vi "GradientSearchCoupling.vi"(0 "System no.":i32=1 min=1 max=4 step=1, 1 "Gradient Scan Names":string[](array[string]), 5 "error in (no error)":errorcluster) -> (19 "error out":errorcluster)   [LabVIEW 2020]
doc: "This VI allows to couple gradient search routines using the FRC command.\nAll changes are sent to the controller by pressing the OK button. If Cancel is selected or the window is closed, nothing will be sent to the controller."
uses:
  <vilib>/Utility/miscctls.llb/LVRowAndColumnTypeDef.ctl
  <vilib>/Utility/cursorutil.llb/Set Cursor (Icon Pict).vi
panel:
  in  "Gradient Search Routine Coupling":string[][](table)
  in  "OK Button":bool
  in  "Cancel Button":bool
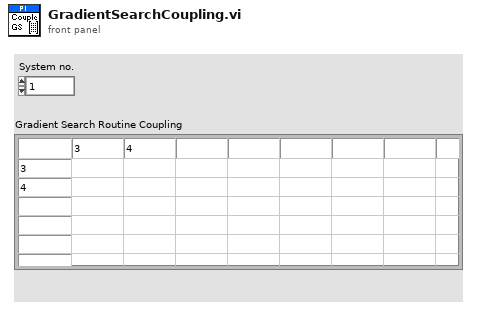
[diagram p1: front panel]
types:
  T1 = typedef "LVRowAndColumnTypeDef.ctl" = cluster{"Row":i32, "Column":i32}
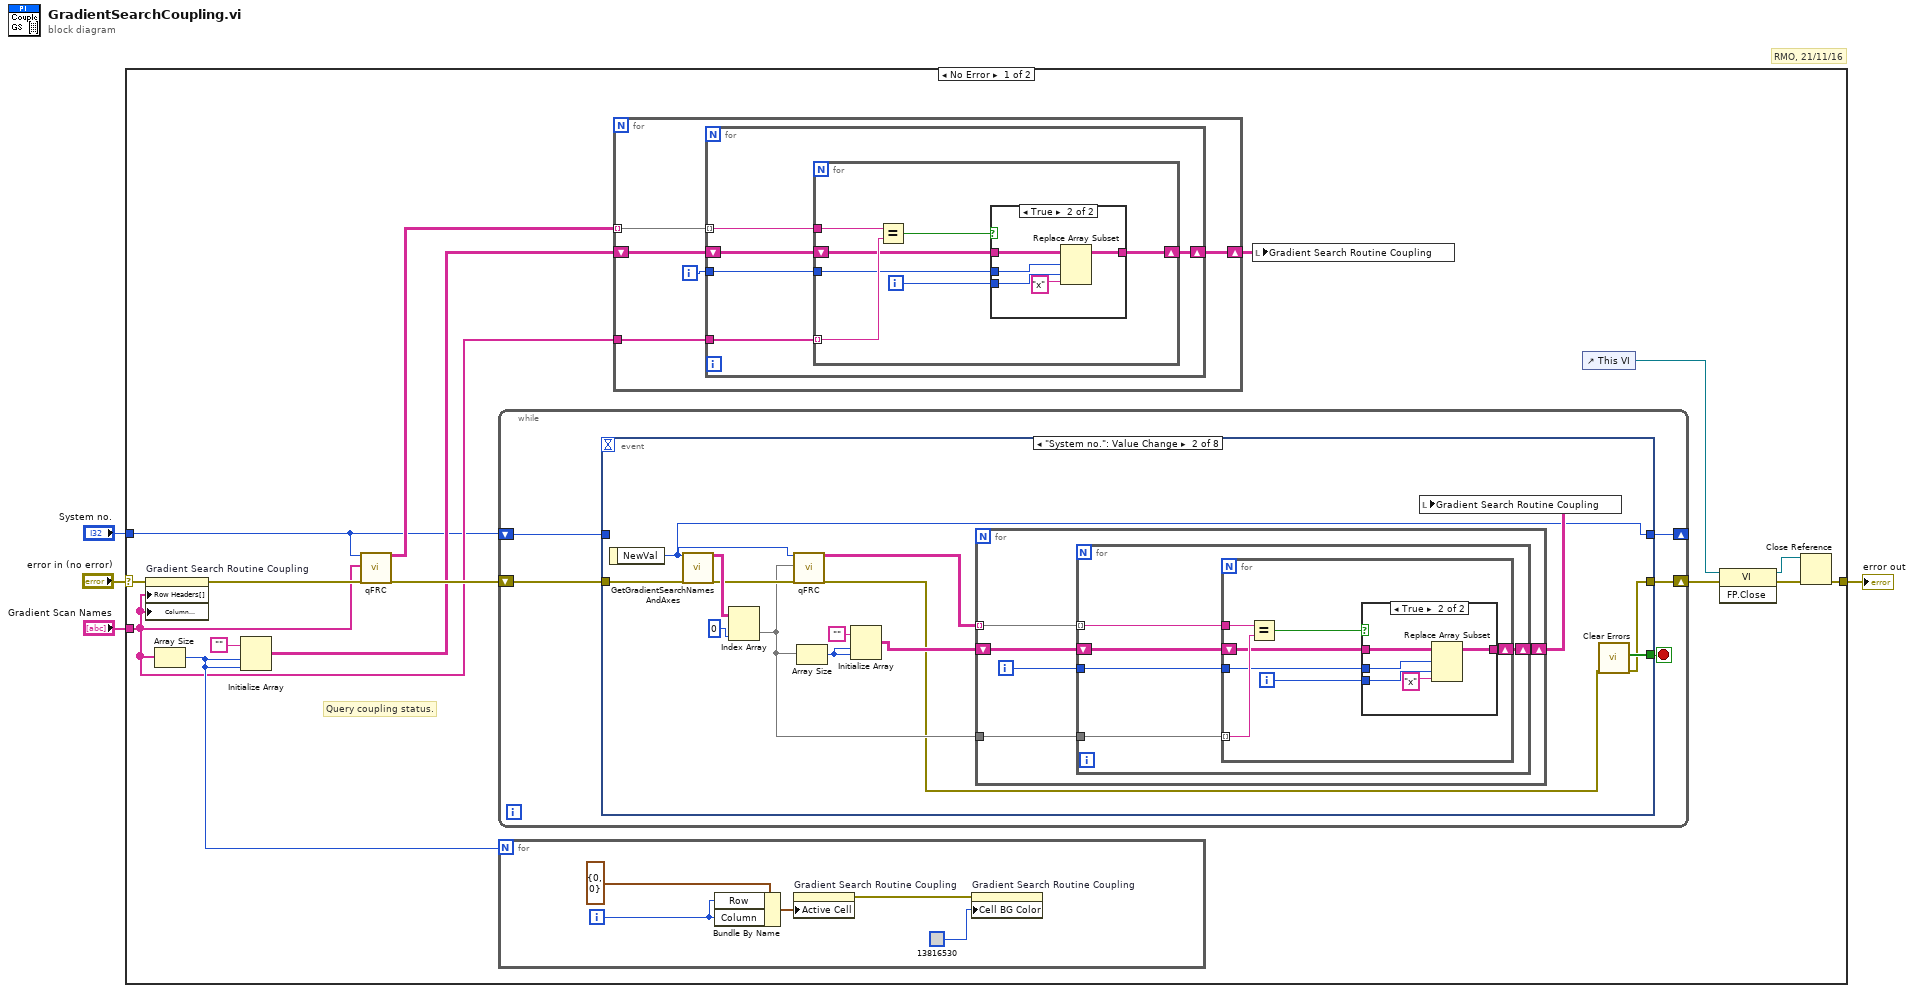
[diagram p0: block diagram]
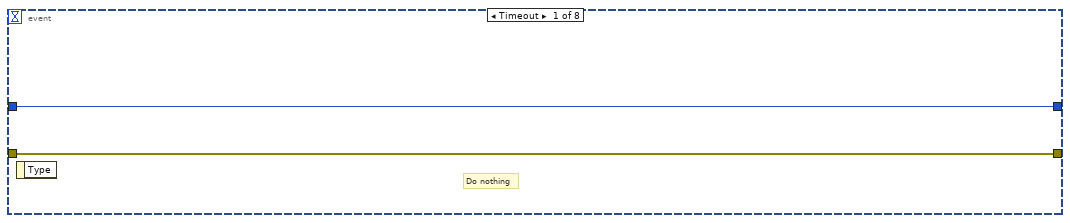
[diagram p3: hidden frame]
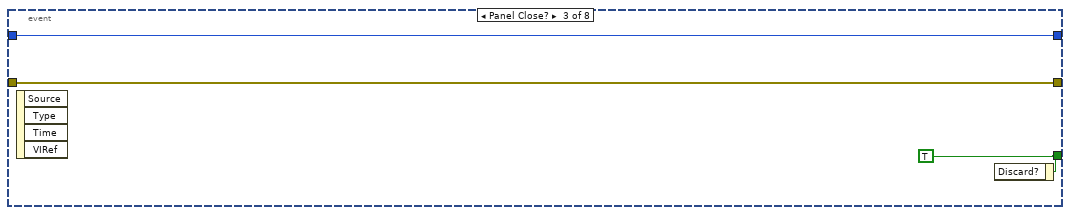
[diagram p5: hidden frame]
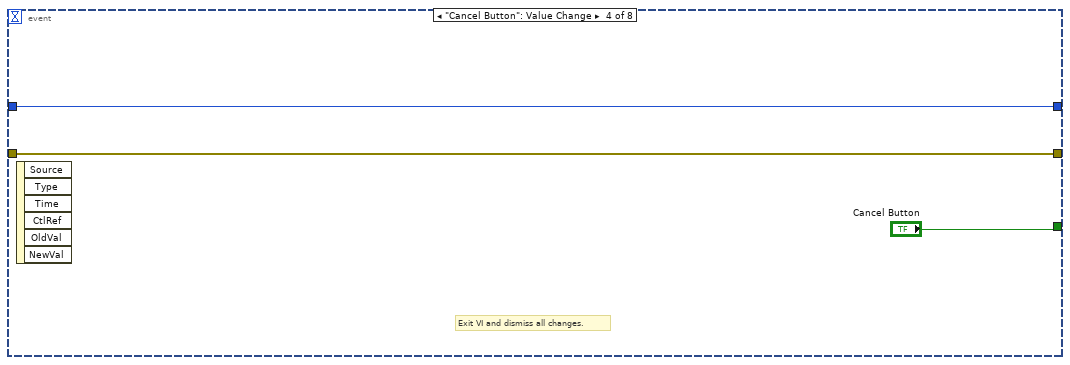
[diagram p6: hidden frame]
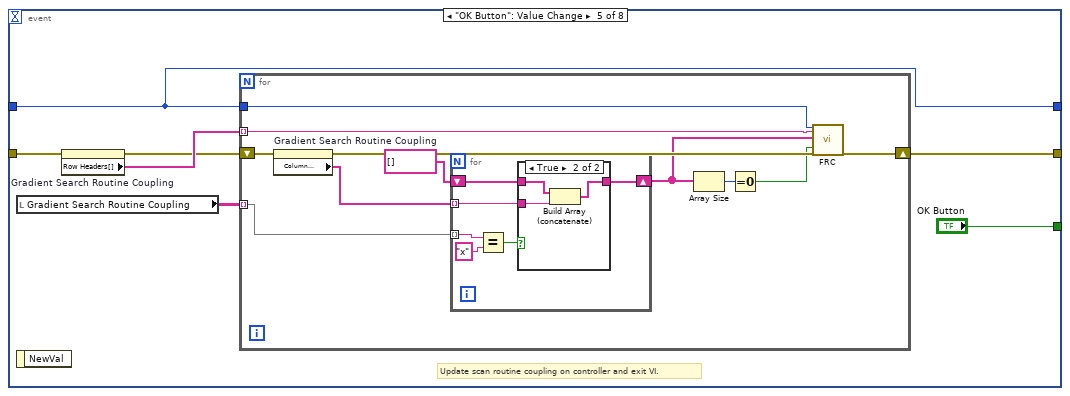
[diagram p7: hidden frame]
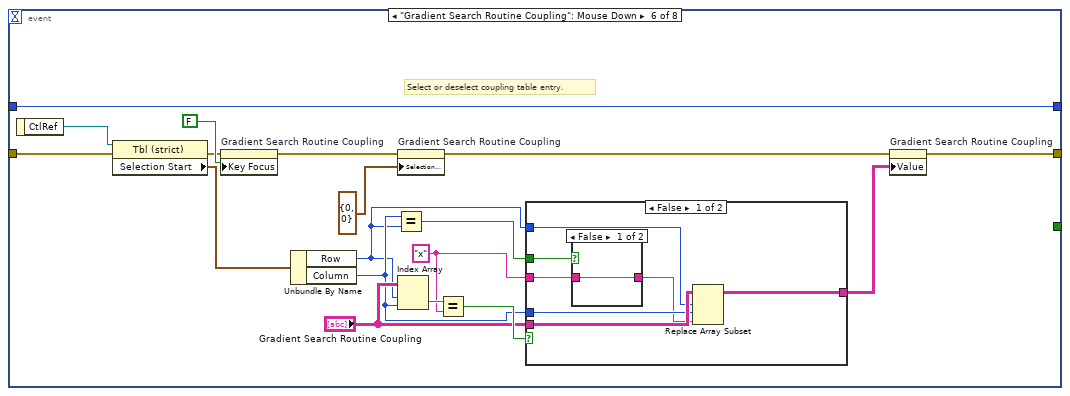
[diagram p9: hidden frame]
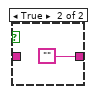
[diagram p10: hidden frame]
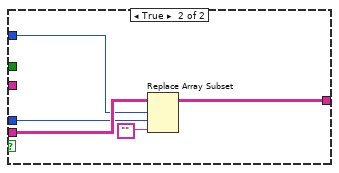
[diagram p11: hidden frame]
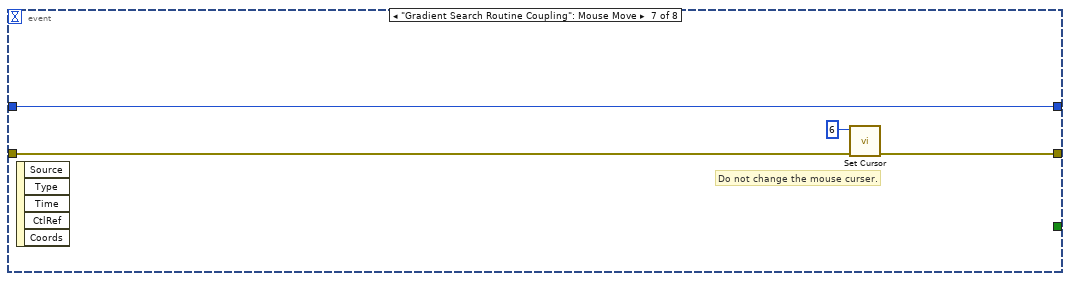
[diagram p12: hidden frame]
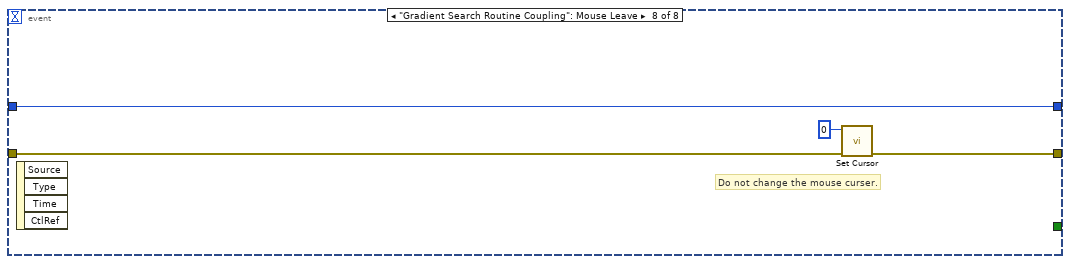
[diagram p13: hidden frame]
diagram:
  # "RMO, 21/11/16"
  n1 = case shown="No Error" "error in (no error)" {
    selector: "error in (no error)" -> [w19 w165]
    tunnel: [w8 w165] -> w4
    tunnel: "Gradient Scan Names" -> [w13 _]
    tunnel: "System no." -> [w10 _]
    frame No Error {
      # "Query coupling status."
      n2 = property on="Gradient Search Routine Coupling" class="Tbl (strict)"(error in=w19, "Row Headers[]"=w13, "Column Headers[]"=w13) -> (error out=w16:errorcluster)  [unwired: 1 in, 1 out]
      n3 = Array Size(array=w13) -> (size(s)=w17:i32)
      n4 = Initialize Array("", w17, w17) -> (w11:string[][])
      n5 = call "qFRC.vi"("System no."=w10, "Routines to query"=w13, "error in"=w16) -> ("Routines coupled"=w14:string[][], "error out"=w15:errorcluster)  [unwired: 1 in, 14 out]
      n6 = while {
        shift-right: [w50] -> w9
        shift-left: w15 -> [w51]
        shift-right: [w48] -> _
        shift-left: w10 -> [w49]
        stop <- w52 stop-if-true
        n7 = event shown="[1] \"System no.\": Value Change" {
          selector: _ -> [_ _ _ _ _ _ _ _]
          dyn-events: _ -> [_ _ _ _ _ _ _ _]
          timeout: _ -> [_ _ _ _ _ _ _ _]
          tunnel: [_ _ w92 "Cancel Button" "OK Button" _ _ _] -> w52
          tunnel: w51 -> [w54 w66 w93 w96 w100 w140 w159 w163]
          tunnel: [w54 w55 w93 w96 w99 w126 w158 w162] -> w50
          tunnel: w49 -> [w53 _ w91 w94 w97 w125 w157 w161]
          tunnel: [w53 w58 w91 w94 w97 w125 w157 w161] -> w48
          event Timeout {
            # "Do nothing"
            n8 = event-data() -> ()  [unwired: 2 out]
          }
          event "System no.": Value Change {
            n9 = event-data() -> ("NewVal"=w58:i32)  [unwired: 1 out]
            n10 = call "GetGradientSearchNamesAndAxes.vi"("System no."=w58, "error in"=w66) -> ("Scan Name, Scan Axis, Step Axis"=w67:string[][], "error out"=w65:errorcluster)  [unwired: 16 out]
            n11 = Index Array(array=w67, index (col)=0 ("index")) -> (element=w59:string[])  [unwired: 1 in]
            n12 = call "qFRC.vi"("System no."=w58, "Routines to query"=w59, "error in"=w65) -> ("Routines coupled"=w63:string[][], "error out"=w56:errorcluster)  [unwired: 1 in, 14 out]
            n13 = Array Size(array=w59) -> (size(s)=w62:i32)
            n14 = Initialize Array("", w62, w62) -> (w60:string[][])
            n15 = for {
              tunnel: w63 -> [w72] mode=indexing
              tunnel: w59 -> [w70]
              shift-right: [w69] -> w64
              shift-left: w60 -> [w71]
              i -> [w68]
              n16 = for {
                tunnel: w72 -> [w76] mode=indexing
                tunnel: w70 -> [w77]
                shift-right: [w74] -> w69
                shift-left: w71 -> [w75]
                tunnel: w68 -> [w73]
                n17 = for {
                  tunnel: w77 -> [w83] mode=indexing
                  tunnel: w76 -> [w84]
                  shift-right: [w78] -> w74
                  shift-left: w75 -> [w80]
                  tunnel: w73 -> [w79]
                  i -> [w81]
                  n18 = Equal?(x=w84, y=w83) -> (x = y?=w82:bool)
                  n19 = case shown="True" w82 {
                    tunnel: w81 -> [_ w86]
                    tunnel: w80 -> [w85 w90]
                    tunnel: w79 -> [_ w87]
                    tunnel: [w85 w88] -> w78
                    frame False {
                    }
                    frame True {
                      n20 = Replace Array Subset(array=w90, new element="x", index (row)=w87, index (col)=w86) -> (w88:string[][])
                    }
                  }
                }
              }
            }
            n21 = local write "Gradient Search Routine Coupling"(w64) -> ()
            n22 = call <vilib>:"Clear Errors.vi"("error in (no error)"=w56) -> ("error out"=w55:errorcluster)  [unwired: 1 in, 5 out]
          }
          event Panel Close? {
            w92 = TRUE
            n23 = event-data() -> ()  [unwired: 5 out]
            n24 = event-data("Discard?"=w92) -> ()  [unwired: 1 in, 1 out]
          }
          event "Cancel Button": Value Change {
            # "Exit VI and dismiss all changes."
            n25 = event-data() -> ()  [unwired: 7 out]
          }
          event "OK Button": Value Change {
            # "Update scan routine coupling on controller and exit VI."
            n26 = local read "Gradient Search Routine Coupling"() -> (w102:string[][])
            n27 = event-data() -> ()  [unwired: 2 out]
            n28 = property on="Gradient Search Routine Coupling" class="Tbl (strict)"(error in=w100) -> (error out=w98:errorcluster, "Row Headers[]"=w101:string[])  [unwired: 1 in, 1 out]
            n29 = for {
              tunnel: w102 -> [w109] mode=indexing
              tunnel: w101 -> [w111] mode=indexing
              tunnel: w97 -> [w112]
              shift-right: [w113] -> w99
              shift-left: w98 -> [w114]
              n30 = property on="Gradient Search Routine Coupling" class="Tbl (strict)"(error in=w114) -> (error out=w108:errorcluster, "Column Headers[]"=w110:string[])  [unwired: 1 in, 1 out]
              n31 = for {
                shift-right: [w115] -> w106
                shift-left: string[] [] -> [w117]
                tunnel: w110 -> [w116] mode=indexing
                tunnel: w109 -> [w120] mode=indexing
                n32 = Equal?(x=w120, y="x") -> (x = y?=w118:bool)
                n33 = case shown="True" w118 {
                  tunnel: w117 -> [w121 w124]
                  tunnel: w116 -> [_ w123]
                  tunnel: [w121 w122] -> w115
                  frame False {
                  }
                  frame True {
                    n34 = Build Array (concatenate)(w124, w123) -> (w122:string[])
                  }
                }
              }
              n35 = Array Size(array=w106) -> (size(s)=w105:i32)
              n36 = Equal To 0?(x=w105) -> (x = 0?=w104:bool)
              n37 = call "FRC.vi"("System no."=w112, "Base routine name"=w111, "Routines to couple to"=w106, "Remove routine coupling?"=w104, "error in"=w108) -> ("error out"=w113:errorcluster)  [unwired: 14 out]
            }
          }
          event "Gradient Search Routine Coupling": Mouse Down {
            w136 = "x" ("y")
            # "Select or deselect coupling table entry."
            n38 = event-data() -> ("CtlRef"=w142:refnum<vi>)  [unwired: 1 out]
            n39 = property class="Tbl (strict)"(reference=w142, error in=w140) -> (error out=w134:errorcluster, "Selection Start"=w141:T1)  [unwired: 1 out]
            n40 = property on="Gradient Search Routine Coupling" class="Tbl (strict)"(error in=w134, "Key Focus"=FALSE) -> (error out=w133:errorcluster)  [unwired: 1 in, 1 out]
            n41 = Unbundle By Name(w141) -> ("Row"=w130:i32, "Column"=w131:i32)
            n42 = Equal?(x=w131, y=w130) -> (x = y?=w129:bool)
            n43 = property on="Gradient Search Routine Coupling" class="Tbl (strict)"(error in=w133, "Selection Start"=T1 {"Row"=0, "Column"=0} ("Edit Position")) -> (error out=w127:errorcluster)  [unwired: 1 in, 1 out]
            n44 = Index Array(array="Gradient Search Routine Coupling", index (row)=w130, index (col)=w131) -> (element=w139:string)
            n45 = Equal?(x=w139, y=w136) -> (x = y?=w138:bool)
            n46 = case shown="False" w138 {
              tunnel: "Gradient Search Routine Coupling" -> [w149 w156]
              tunnel: w130 -> [w148 w155]
              tunnel: w131 -> [w147 w154]
              tunnel: w136 -> [w144 _]
              tunnel: [w146 w152] -> w128
              tunnel: w129 -> [w145 _]
              frame False {
                n47 = case shown="False" w145 {
                  tunnel: w144 -> [w150 _]
                  tunnel: [w150 ""] -> w143
                  frame False {
                  }
                  frame True {
                  }
                }
                n48 = Replace Array Subset(array=w149, new element=w143, index (row)=w148, index (col)=w147) -> (w146:string[][])
              }
              frame True {
                n49 = Replace Array Subset(array=w156, new element="", index (row)=w155, index (col)=w154) -> (w152:string[][])
              }
            }
            n50 = property on="Gradient Search Routine Coupling" class="Tbl (strict)"(error in=w127, "Value"=w128) -> (error out=w126:errorcluster)  [unwired: 1 in, 1 out]
          }
          event "Gradient Search Routine Coupling": Mouse Move {
            # "Do not change the mouse curser."
            n51 = event-data() -> ()  [unwired: 6 out]
            n52 = call-poly <vilib>:"Set Cursor.vi"("error in (no error)"=w159, "icon"=u16 6) -> ("error out"=w158:errorcluster)  [unwired: 1 in, 8 out]
          }
          event "Gradient Search Routine Coupling": Mouse Leave {
            # "Do not change the mouse curser."
            n53 = event-data() -> ()  [unwired: 5 out]
            n54 = call-poly <vilib>:"Set Cursor.vi"("error in (no error)"=w163, "icon"=u16 0) -> ("error out"=w162:errorcluster)  [unwired: 1 in, 8 out]
          }
        }
      }
      n55 = for {
        N: w17 -> [_]
        i -> [w44]
        n56 = Bundle By Name(cluster=T1 {"Row"=0, "Column"=0} ("Active Cell:Active Cell"), "Row"=w44, "Column"=w44) -> (w43:T1)
        n57 = property on="Gradient Search Routine Coupling" class="Tbl (strict)"("Active Cell"=w43) -> (error out=w47:errorcluster)  [unwired: 2 in, 1 out]
        n58 = property on="Gradient Search Routine Coupling" class="Tbl (strict)"(error in=w47, "Cell BG Color"=u32 13816530) -> ()  [unwired: 1 in, 2 out]
      }
      n59 = for {
        tunnel: w14 -> [w24] mode=indexing
        tunnel: w13 -> [w22]
        shift-right: [w21] -> w12
        shift-left: w11 -> [w23]
        i -> [w20]
        n60 = for {
          tunnel: w24 -> [w28] mode=indexing
          tunnel: w22 -> [w29]
          shift-right: [w26] -> w21
          shift-left: w23 -> [w27]
          tunnel: w20 -> [w25]
          n61 = for {
            tunnel: w29 -> [w35] mode=indexing
            tunnel: w28 -> [w36]
            shift-right: [w30] -> w26
            shift-left: w27 -> [w32]
            tunnel: w25 -> [w31]
            i -> [w33]
            n62 = Equal?(x=w36, y=w35) -> (x = y?=w34:bool)
            n63 = case shown="True" w34 {
              tunnel: w33 -> [_ w38]
              tunnel: w32 -> [w37 w42]
              tunnel: w31 -> [_ w39]
              tunnel: [w37 w40] -> w30
              frame False {
              }
              frame True {
                n64 = Replace Array Subset(array=w42, new element="x", index (row)=w39, index (col)=w38) -> (w40:string[][])
              }
            }
          }
        }
      }
      n65 = local write "Gradient Search Routine Coupling"(w12) -> ()
      n66 = control-ref of="This VI"() -> (w5:refnum<vi>)
      n67 = invoke class="VI" method="FP.Close"(reference=w5, error in=w9) -> (reference out=w7:refnum<vi>, error out=w6:errorcluster)  [unwired: 1 in, 1 out]
      n68 = Close Reference(reference=w7, error in (no error)=w6) -> (error out=w8:errorcluster)
    }
    frame Error {
    }
  }
  "error out" <- w4
